vi "Read Cache.vi"(8 "error in (no error)":errorcluster, 11 "navX Registry Cache in":refnum<class "navX Registry Cache.lvclass">) -> (0 "error out":errorcluster, 2 "Registry Cache out":u8[](array[numeric]), 3 "navX Registry Cache out":refnum<class "navX Registry Cache.lvclass">)   [LabVIEW 2015, in "navX Library v3.lvlib" / "navX Registry Cache.lvclass"]
uses:
  navX Registry Cache.lvclass
  navX Registry Cache.lvclass/navX Registry Cache.ctl
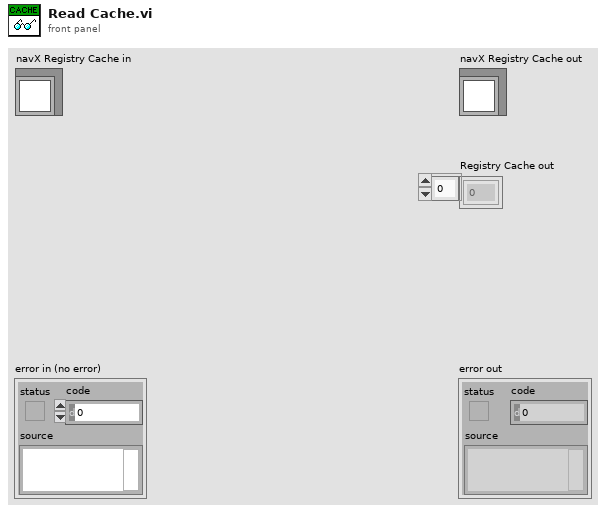
[diagram p1: front panel]
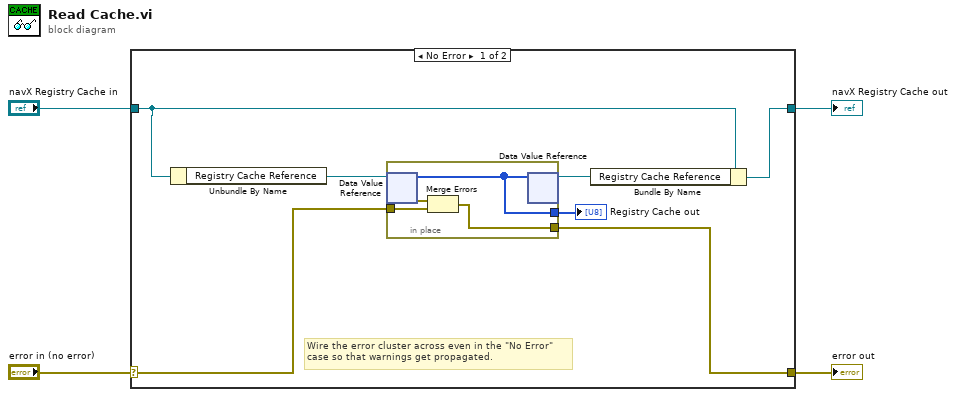
[diagram p0: block diagram]
diagram:
  n1 = case shown="No Error" "error in (no error)" {
    selector: "error in (no error)" -> [w6 w17]
    tunnel: [w5 w17] -> w3
    tunnel: [w8 w16] -> w1
    tunnel: "navX Registry Cache in" -> [w9 w16]
    frame No Error {
      # "Wire the error cluster across even in the \"No Error\"\ncase so that warnings get propagated."
      n2 = Unbundle By Name(w9) -> ("Registry Cache Reference"=w10:refnum<data-value>)
      n3 = in-place {
        in-place-border: [w15] -> w7
        in-place-border: w6 -> [w13]
        in-place-border: [w12] -> w5
        n4 = in-place-dvr #1(w10) -> (w15:u8[], w14:errorcluster)
        n5 = Merge Errors(w14, w13) -> (w12:errorcluster)
        n6 = in-place-dvr #1(w15) -> (w11:refnum<data-value>)  [unwired: 1 out]
      }
      "Registry Cache out" <- w7
      n7 = Bundle By Name(cluster=w9, "Registry Cache Reference"=w11) -> (w8:refnum<class "navX Registry Cache.lvclass">)
    }
    frame Error {
    }
  }
  "error out" <- w3
  "navX Registry Cache out" <- w1
